vi "3_1.vi"() -> ()   [LabVIEW 2019]
panel:
  out "# iteraction":dbl
  in  "Numer to match":dbl=50.0 min=0.0 max=10000.0 step=1.0 format="%#.0f"
  out "Current\nnumber":dbl
  # "*numeric indicator*"
  # "*numeric control*\n\nData control\n     Default =50\n      Min=0\n      Max=10000\n      Inc=1\n\nPrecision=0"
  # "Presicion=0"
  # "*numeric indactor*\n\n   Presicion=0"
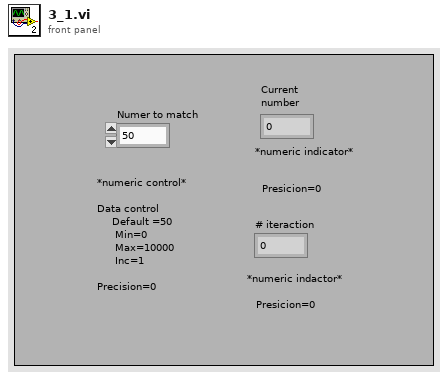
[diagram p1: front panel]
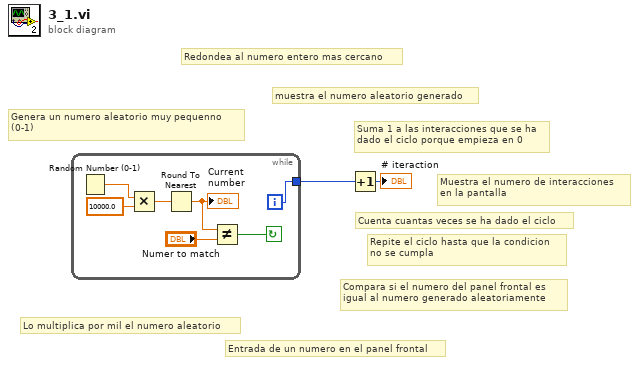
[diagram p0: block diagram]
diagram:
  # "Muestra el numero de interacciones\nen la pantalla"
  # "Suma 1 a las interacciones que se ha\ndado el ciclo porque empieza en 0"
  # "Cuenta cuantas veces se ha dado el ciclo"
  # "Repite el ciclo hasta que la condicion\nno se cumpla"
  # "Compara si el numero del panel frontal es \nigual al numero generado aleatoriamente"
  # "Entrada de un numero en el panel frontal"
  # "Redondea al numero entero mas cercano"
  # "muestra el numero aleatorio generado"
  # "Lo multiplica por mil el numero aleatorio"
  # "Genera un numero aleatorio muy pequenno\n(0-1)"
  n1 = while {
    tunnel: [w3] -> w2
    i -> [w3]
    stop <- w4 continue-if-true
    n2 = Random Number (0-1)() -> (number: 0 to 1=w8:dbl)
    n3 = Multiply(x=w8, y=10000.0) -> (x*y=w7:dbl)
    n4 = Round To Nearest(number=w7) -> (nearest integer value=w6:dbl)
    "Current\nnumber" <- w6
    n5 = Not Equal?(x=w6, y="Numer to match") -> (x != y?=w4:bool)
  }
  n6 = Increment(x=w2) -> (x+1=→"# iteraction":i32)
